vi "Pockels task.vi"(8 "error in (no error)":errorcluster, 11 "Setup/Logging queue element":T2={"Imaging Protocol"=enum."Live Imaging", "Number of Trials"=0, "Frame Size"=512, "# Averaged frames"=0, "Dwell time (us)"=0.0, "Index of Z-plane"=0, "Timelapse?"=FALSE, "Logging process is active"=FALSE, "Speed logging enabled"=FALSE, "tdms file ref"=refnum, "path"=path "", "Trial Number"=0, "Expected # points acquired"=FALSE, "Manually stopped"=FALSE, "Ch0 data"=[], "Ch1 data"=[], "Ref Data"=[], "Last trial"=FALSE, "Ref Dwell time (us)"=0.0, "# Ref Averaged frames"=0, "Ref X Length"=0, "Ref Y Length"=0, "Points acquired"={"Ch0 last trial"=0, "Ch1 last trial"=0, "All trials"=0}} {"Ref Dwell time (us)" format="%#.6g"; "Frame Size" items=["100X100"=100, "128X128"=128, "200X200"=200, "256X256"=256, "512X512"=512, "1024x1024"=1024, "2048x2048"=2048]; "Dwell time (us)" format="%#.6g"}) -> (0 "error out":errorcluster)   [LabVIEW 2017]
uses:
  Typedefs/Logging queue element.ctl
  Typedefs/Imaging Protocols enum.ctl
  Typedefs/Frame Size.ctl
  Typedefs/Acquired points count.ctl
  Typedefs/Triggered tasks cluster.ctl
  Globals/gl_Triggering globals.vi
panel:
  out "Info":T1 {"Sampling period (us)" format="%#_6f"; "Data lenght (ms)" format="%#_6f"}
  out "# of DO points":i32
  out "Digital Waveform Graph":digitaldata(graph)
  out "Waveform Graph":dbl[](graph)
  out "# of AO points":i32
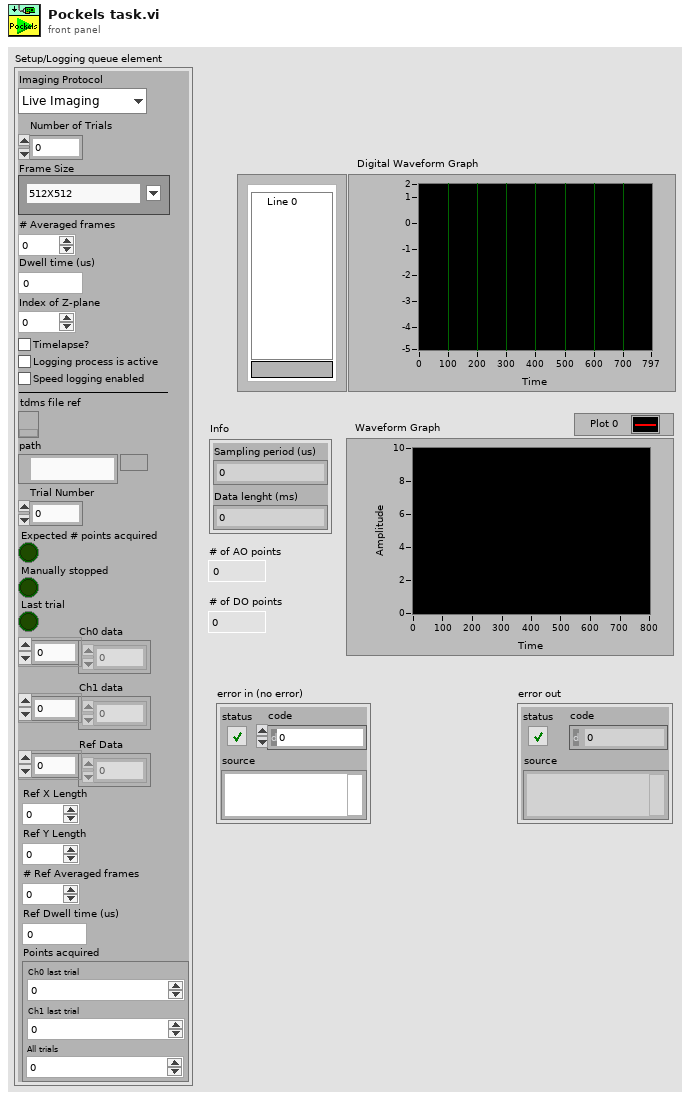
[diagram p1: front panel]
types:
  T1 = cluster{"Sampling period (us)":dbl, "Data lenght (ms)":dbl}
  T2 = typedef "Logging queue element.ctl" = cluster{"Imaging Protocol":T3, "Number of Trials":u16, "Frame Size":T4, "# Averaged frames":u16, "Dwell time (us)":dbl, "Index of Z-plane":i32, "Timelapse?":bool, "Logging process is active":bool, "Speed logging enabled":bool, "tdms file ref":refnum<k34>, "path":path, "Trial Number":i32, "Expected # points acquired":bool, "Manually stopped":bool, "Ch0 data":u32[], "Ch1 data":u32[], "Ref Data":u32[], "Last trial":bool, "Ref Dwell time (us)":dbl, "# Ref Averaged frames":u16, "Ref X Length":u16, "Ref Y Length":u16, "Points acquired":T5}
  T3 = typedef "Imaging Protocols enum.ctl" = enum16{"AOL Z-Stack", "Motor Z Stack", "Functional Acquisition", "Single Plane Acquisition", "Volume Acquisition", "Live Imaging", "Live Plane Imaging", "Live Volume Imaging"}
  T4 = typedef "Frame Size.ctl" = u16
  T5 = typedef "Acquired points count.ctl" = cluster{"Ch0 last trial":u64, "Ch1 last trial":u64, "All trials":u64}
  T6 = typedef "Triggered tasks cluster.ctl" = cluster{"DO task-Encoder trigger":refnum<k21>, "AO Task-Pockels modulation":refnum<k21>, "Counter Clock Task":refnum<k21>}
  T7 = cluster{"Sampling period (us)":dbl, "Data length (ms)":dbl}
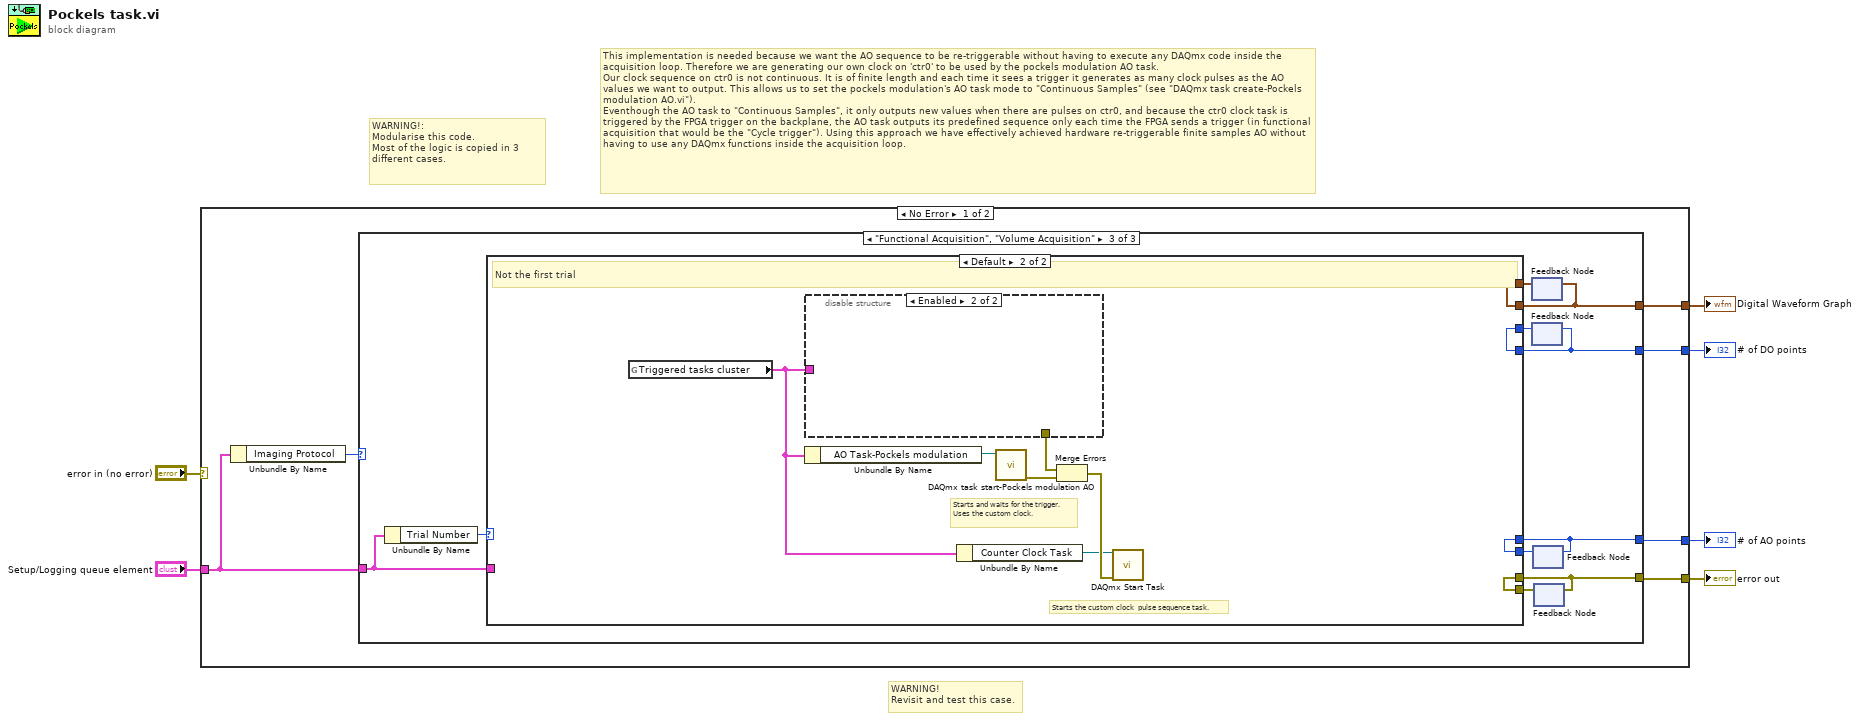
[diagram p0: block diagram]
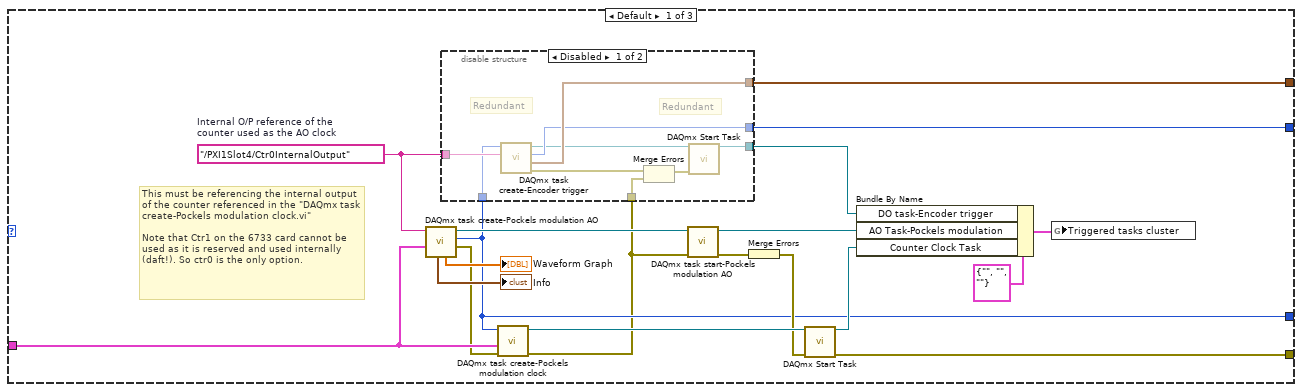
[diagram p2: hidden frame]
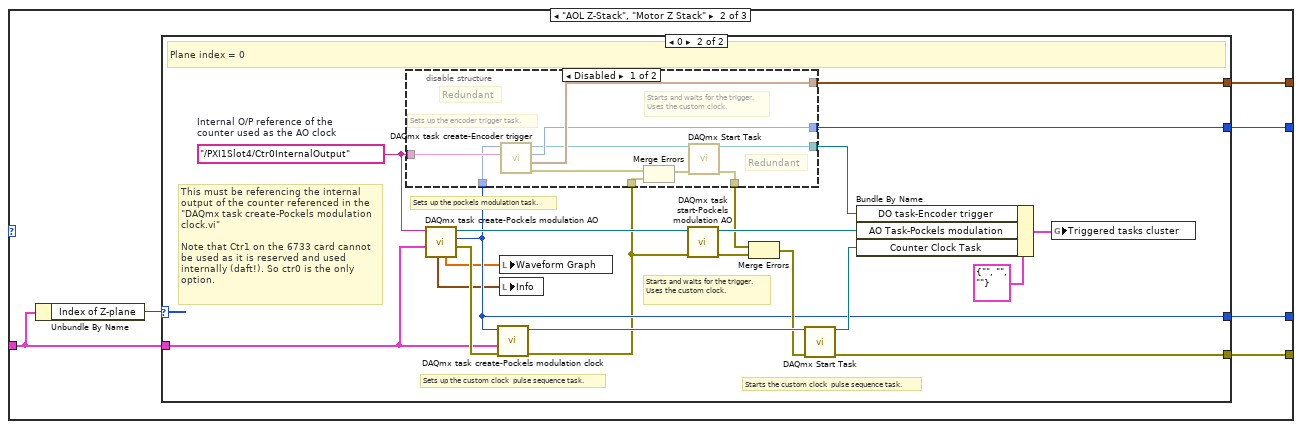
[diagram p4: hidden frame]
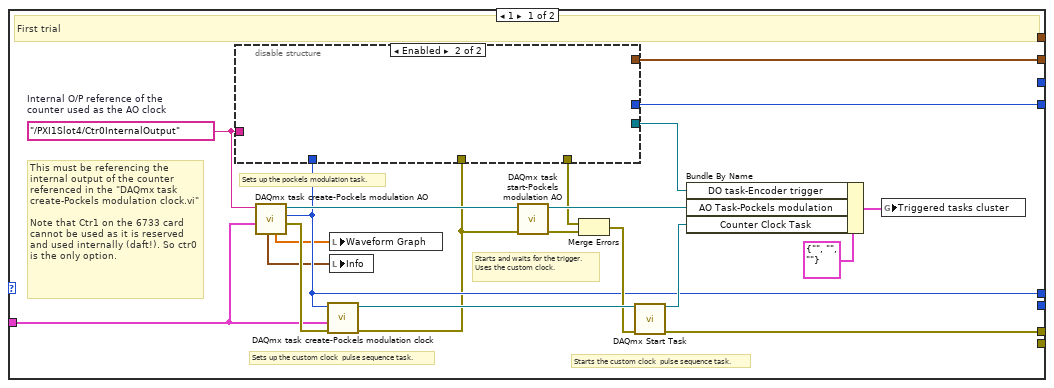
[diagram p7: hidden frame]
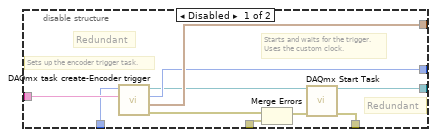
[diagram p8: hidden frame]
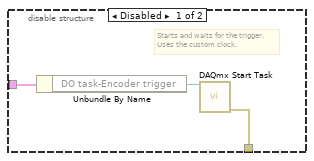
[diagram p9: hidden frame]
diagram:
  # "WARNING!\nRevisit and test this case."
  # "WARNING!:\nModularise this code.\nMost of the logic is copied in 3 different cases."
  # "This implementation is needed because we want the AO sequence to be re-triggerable without having to execute any DAQmx code inside the acquisition loop. Therefore we are generating our own clock on 'ctr0' to be used by the pockels modulation AO task.\nOur clock sequence on ctr0 is not continuous. It is of finite length and each time it sees a trigger it generates as many clock pulses as the AO values we want to output. This allows us to set the pockels modulation's AO task mode to \"Continuous Samples\" (see \"DAQmx task create-Pockels modulation AO.vi\").\nEventhough the AO task to \"Continuous Samples\", it only outputs new values when there are pulses on ctr0, and because the ctr0 clock task is triggered by the FPGA trigger on the backplane, the AO task outputs its predefined sequence only each time the FPGA sends a trigger (in functional acquisition that would be the \"Cycle trigger\"). Using this approach we have effectively achieved hardware re-triggerable finite samples AO without having to use any DAQmx functions inside the acquisition loop."
  n1 = case shown="No Error" "error in (no error)" {
    selector: "error in (no error)" -> [_ w130]
    tunnel: [w12 w130] -> w5
    tunnel: [w9 _] -> w4
    tunnel: [w11 _] -> w3
    tunnel: "Setup/Logging queue element" -> [w8 _]
    tunnel: [w10 _] -> w2
    frame No Error {
      n2 = Unbundle By Name(w8) -> ("Imaging Protocol"=w7:T3)
      n3 = case shown="\"Functional Acquisition\", \"Volume Acquisition\"" w7 {
        tunnel: [w28 w46 w82] -> w12
        tunnel: [w25 w45 w84] -> w11
        tunnel: [w24 w44 w80] -> w10
        tunnel: w8 -> [w18 w42 w86]
        tunnel: [w14 w43 w81] -> w9
        frame Default {
          w17 = tag "/PXI1Slot4/Ctr0InternalOutput"  # Internal O/P reference of the  counter used as the AO clock
          # "This must be referencing the internal output of the counter referenced in the \"DAQmx task create-Pockels modulation clock.vi\"\n\nNote that Ctr1 on the 6733 card cannot be used as it is reserved and used internally (daft!). So ctr0 is the only option."
          n4 = call "DAQmx task create-Pockels modulation AO.vi"("Setup/Logging queue element"=w18, "Internal O/P reference of the \ncounter used as the AO clock"=w17) -> ("error out"=w15:errorcluster, "Data length (points)"=w14:i32, "Pockels modulation AO task"=w20:refnum<k21>, "Info"=→"Info":T7, "Pockels modulation data out"=→"Waveform Graph":dbl[])  [unwired: 5 in]
          n5 = call "DAQmx task create-Pockels modulation clock.vi"("error in"=w15, "Setup/Logging queue element"=w18, "Data length"=w14) -> ("error out"=w13:errorcluster, "Refnum out"=w22:refnum<k21>)  [unwired: 7 in]
          n6 = disable-structure shown="Disabled" {
            disable-tunnel: [w40 _] -> w27
            disable-tunnel: [w39 _] -> w25
            disable-tunnel: [w38 _] -> w24
            disable-tunnel: w17 -> [w37 _]
            disable-tunnel: w14 -> [w35 _]
            disable-tunnel: w13 -> [w34 _]
            frame Disabled {
              # "Redundant"
              # "Redundant"
              n7 = call "DAQmx task create-Encoder trigger.vi"("Internal O/P reference of the \ncounter used as the AO clock"=w37, "Data length"=w35) -> ("error out"=w33:errorcluster, "Encoder trigger DO sequence"=w39:digitaldata, "# points in output waveform"=w38:i32, "Refnum out"=w32:refnum<k21>)  [unwired: 6 in]
              n8 = Merge Errors(w33, w34) -> (w36:errorcluster)
              n9 = call <vilib>:"DAQmx Start Task.vi"("task/channels in"=w32, "error in"=w36) -> ("task out"=w40:refnum<k21>)  [unwired: 12 in, 1 out]
            }
            frame Enabled {
            }
          }
          n10 = call "DAQmx task start-Pockels modulation AO.vi"("error in (no error)"=w13, "Pockels modulation AO task in"=w20) -> ("error out"=w23:errorcluster, "Pockels modulation AO task out"=w26:refnum<k21>)  [unwired: 8 in]
          n11 = Merge Errors(w23) -> (w21:errorcluster)
          n12 = call <vilib>:"DAQmx Start Task.vi"("task/channels in"=w22, "error in"=w21) -> ("task out"=w29:refnum<k21>, "error out"=w28:errorcluster)  [unwired: 12 in]
          n13 = Bundle By Name(cluster=T6 {"DO task-Encoder trigger"="", "AO Task-Pockels modulation"="", "Counter Clock Task"=""}, "DO task-Encoder trigger"=w27, "AO Task-Pockels modulation"=w26, "Counter Clock Task"=w29) -> (w31:T6)
          n14 = global write "gl_Triggering globals.vi" "Triggered tasks cluster"(w31) -> ()
        }
        frame "AOL Z-Stack", "Motor Z Stack" {
          n15 = Unbundle By Name(w42) -> ("Index of Z-plane"=w41:i32)
          n16 = case shown="0" w41 {
            tunnel: [_ w63] -> w46
            tunnel: [_ w60] -> w45
            tunnel: [_ w59] -> w44
            tunnel: [_ w52] -> w43
            tunnel: w42 -> [_ w50]
            frame Default {
              # "Plane index is other than zero"
            }
            frame 0 {
              w54 = tag "/PXI1Slot4/Ctr0InternalOutput"  # Internal O/P reference of the  counter used as the AO clock
              # "Sets up the pockels modulation task."
              # "Sets up the custom clock  pulse sequence task."
              # "Starts the custom clock  pulse sequence task."
              # "Starts and waits for the trigger.\nUses the custom clock."
              # "This must be referencing the internal output of the counter referenced in the \"DAQmx task create-Pockels modulation clock.vi\"\n\nNote that Ctr1 on the 6733 card cannot be used as it is reserved and used internally (daft!). So ctr0 is the only option."
              # "Plane index = 0"
              n17 = call "DAQmx task create-Pockels modulation AO.vi"("Setup/Logging queue element"=w50, "Internal O/P reference of the \ncounter used as the AO clock"=w54) -> ("error out"=w53:errorcluster, "Data length (points)"=w52:i32, "Pockels modulation AO task"=w55:refnum<k21>, "Info"=w49:T7, "Pockels modulation data out"=w48:dbl[])  [unwired: 5 in]
              n18 = call "DAQmx task create-Pockels modulation clock.vi"("error in"=w53, "Setup/Logging queue element"=w50, "Data length"=w52) -> ("error out"=w51:errorcluster, "Refnum out"=w57:refnum<k21>)  [unwired: 7 in]
              n19 = disable-structure shown="Disabled" {
                disable-tunnel: [w76 _] -> w62
                disable-tunnel: [w75 _] -> w60
                disable-tunnel: [w74 _] -> w59
                disable-tunnel: w54 -> [w73 _]
                disable-tunnel: w52 -> [w71 _]
                disable-tunnel: w51 -> [w70 _]
                disable-tunnel: [w67 _] -> w47
                frame Disabled {
                  # "Redundant"
                  # "Redundant"
                  # "Sets up the encoder trigger task."
                  # "Starts and waits for the trigger.\nUses the custom clock."
                  n20 = call "DAQmx task create-Encoder trigger.vi"("Internal O/P reference of the \ncounter used as the AO clock"=w73, "Data length"=w71) -> ("error out"=w69:errorcluster, "Encoder trigger DO sequence"=w75:digitaldata, "# points in output waveform"=w74:i32, "Refnum out"=w68:refnum<k21>)  [unwired: 6 in]
                  n21 = Merge Errors(w69, w70) -> (w72:errorcluster)
                  n22 = call <vilib>:"DAQmx Start Task.vi"("task/channels in"=w68, "error in"=w72) -> ("task out"=w76:refnum<k21>, "error out"=w67:errorcluster)  [unwired: 12 in]
                }
                frame Enabled {
                }
              }
              n23 = local write "Waveform Graph"(w48) -> ()
              n24 = local write "Info"(w49) -> ()
              n25 = call "DAQmx task start-Pockels modulation AO.vi"("error in (no error)"=w51, "Pockels modulation AO task in"=w55) -> ("error out"=w58:errorcluster, "Pockels modulation AO task out"=w61:refnum<k21>)  [unwired: 8 in]
              n26 = Merge Errors(w47, w58) -> (w56:errorcluster)
              n27 = call <vilib>:"DAQmx Start Task.vi"("task/channels in"=w57, "error in"=w56) -> ("task out"=w64:refnum<k21>, "error out"=w63:errorcluster)  [unwired: 12 in]
              n28 = Bundle By Name(cluster=T6 {"DO task-Encoder trigger"="", "AO Task-Pockels modulation"="", "Counter Clock Task"=""}, "DO task-Encoder trigger"=w62, "AO Task-Pockels modulation"=w61, "Counter Clock Task"=w64) -> (w66:T6)
              n29 = global write "gl_Triggering globals.vi" "Triggered tasks cluster"(w66) -> ()
            }
          }
        }
        frame "Functional Acquisition", "Volume Acquisition" {
          n30 = Unbundle By Name(w86) -> ("Trial Number"=w85:i32)
          n31 = feedback #1() -> (w83:digitaldata)  [unwired: 1 in]
          n32 = feedback #2() -> (w79:i32)  [unwired: 1 in]
          n33 = feedback #3() -> (w78:i32)  [unwired: 1 in]
          n34 = feedback #4() -> (w77:errorcluster)  [unwired: 1 in]
          n35 = case shown="Default" w85 {
            tunnel: [w103 w120] -> w82
            tunnel: [w100 w123] -> w84
            tunnel: [w99 w122] -> w80
            tunnel: [w92 w121] -> w81
            tunnel: w86 -> [w90 _]
            tunnel: w83 -> [_ w123]
            tunnel: w79 -> [_ w122]
            tunnel: w78 -> [_ w121]
            tunnel: w77 -> [_ w120]
            frame 1 {
              w94 = tag "/PXI1Slot4/Ctr0InternalOutput"  # Internal O/P reference of the  counter used as the AO clock
              # "Sets up the pockels modulation task."
              # "Sets up the custom clock  pulse sequence task."
              # "Starts the custom clock  pulse sequence task."
              # "Starts and waits for the trigger.\nUses the custom clock."
              # "This must be referencing the internal output of the counter referenced in the \"DAQmx task create-Pockels modulation clock.vi\"\n\nNote that Ctr1 on the 6733 card cannot be used as it is reserved and used internally (daft!). So ctr0 is the only option."
              # "First trial"
              n36 = call "DAQmx task create-Pockels modulation AO.vi"("Setup/Logging queue element"=w90, "Internal O/P reference of the \ncounter used as the AO clock"=w94) -> ("error out"=w93:errorcluster, "Data length (points)"=w92:i32, "Pockels modulation AO task"=w95:refnum<k21>, "Info"=w89:T7, "Pockels modulation data out"=w88:dbl[])  [unwired: 5 in]
              n37 = call "DAQmx task create-Pockels modulation clock.vi"("error in"=w93, "Setup/Logging queue element"=w90, "Data length"=w92) -> ("error out"=w91:errorcluster, "Refnum out"=w97:refnum<k21>)  [unwired: 7 in]
              n38 = disable-structure shown="Enabled" {
                disable-tunnel: [w116 _] -> w102
                disable-tunnel: [w115 _] -> w100
                disable-tunnel: [w114 _] -> w99
                disable-tunnel: w94 -> [w113 _]
                disable-tunnel: w92 -> [w111 _]
                disable-tunnel: w91 -> [w110 _]
                disable-tunnel: [w107 _] -> w87
                frame Disabled {
                  # "Redundant"
                  # "Redundant"
                  # "Sets up the encoder trigger task."
                  # "Starts and waits for the trigger.\nUses the custom clock."
                  n39 = call "DAQmx task create-Encoder trigger.vi"("Internal O/P reference of the \ncounter used as the AO clock"=w113, "Data length"=w111) -> ("error out"=w109:errorcluster, "Encoder trigger DO sequence"=w115:digitaldata, "# points in output waveform"=w114:i32, "Refnum out"=w108:refnum<k21>)  [unwired: 6 in]
                  n40 = Merge Errors(w109, w110) -> (w112:errorcluster)
                  n41 = call <vilib>:"DAQmx Start Task.vi"("task/channels in"=w108, "error in"=w112) -> ("task out"=w116:refnum<k21>, "error out"=w107:errorcluster)  [unwired: 12 in]
                }
                frame Enabled {
                }
              }
              n42 = local write "Waveform Graph"(w88) -> ()
              n43 = local write "Info"(w89) -> ()
              n44 = call "DAQmx task start-Pockels modulation AO.vi"("error in (no error)"=w91, "Pockels modulation AO task in"=w95) -> ("error out"=w98:errorcluster, "Pockels modulation AO task out"=w101:refnum<k21>)  [unwired: 8 in]
              n45 = Merge Errors(w87, w98) -> (w96:errorcluster)
              n46 = call <vilib>:"DAQmx Start Task.vi"("task/channels in"=w97, "error in"=w96) -> ("task out"=w104:refnum<k21>, "error out"=w103:errorcluster)  [unwired: 12 in]
              n47 = Bundle By Name(cluster=T6 {"DO task-Encoder trigger"="", "AO Task-Pockels modulation"="", "Counter Clock Task"=""}, "DO task-Encoder trigger"=w102, "AO Task-Pockels modulation"=w101, "Counter Clock Task"=w104) -> (w106:T6)
              n48 = global write "gl_Triggering globals.vi" "Triggered tasks cluster"(w106) -> ()
            }
            frame Default {
              # "Starts the custom clock  pulse sequence task."
              # "Starts and waits for the trigger.\nUses the custom clock."
              # "Not the first trial"
              n49 = global read "gl_Triggering globals.vi" "Triggered tasks cluster"() -> (w117:T6)
              n50 = Unbundle By Name(w117) -> ("AO Task-Pockels modulation"=w119:refnum<k21>)
              n51 = disable-structure shown="Enabled" {
                disable-tunnel: [w129 _] -> w124
                disable-tunnel: w117 -> [w127 _]
                frame Disabled {
                  # "Starts and waits for the trigger.\nUses the custom clock."
                  n52 = Unbundle By Name(w127) -> ("DO task-Encoder trigger"=w128:refnum<k21>)
                  n53 = call <vilib>:"DAQmx Start Task.vi"("task/channels in"=w128) -> ("error out"=w129:errorcluster)  [unwired: 13 in, 1 out]
                }
                frame Enabled {
                }
              }
              n54 = Unbundle By Name(w117) -> ("Counter Clock Task"=w118:refnum<k21>)
              n55 = call "DAQmx task start-Pockels modulation AO.vi"("Pockels modulation AO task in"=w119) -> ("error out"=w126:errorcluster)  [unwired: 9 in, 1 out]
              n56 = Merge Errors(w124, w126) -> (w125:errorcluster)
              n57 = call <vilib>:"DAQmx Start Task.vi"("task/channels in"=w118, "error in"=w125) -> ()  [unwired: 12 in, 2 out]
            }
          }
          n58 = feedback-in #1(w84) -> ()
          n59 = feedback-in #2(w80) -> ()
          n60 = feedback-in #3(w81) -> ()
          n61 = feedback-in #4(w82) -> ()
        }
      }
    }
    frame Error {
    }
  }
  "error out" <- w5
  "# of AO points" <- w4
  "Digital Waveform Graph" <- w3
  "# of DO points" <- w2
